vi "Teleop_TwistandDrive.vi"(9 "Joy Drive Input":dbl, 10 "Deadband X Value":dbl, 11 "Joy Twist Input":dbl) -> (3 "Twist Output":dbl[](array[numeric]))   [LabVIEW 2017]
panel:
  out "XY Graph":cluster{dbl[], dbl[]}(graph)
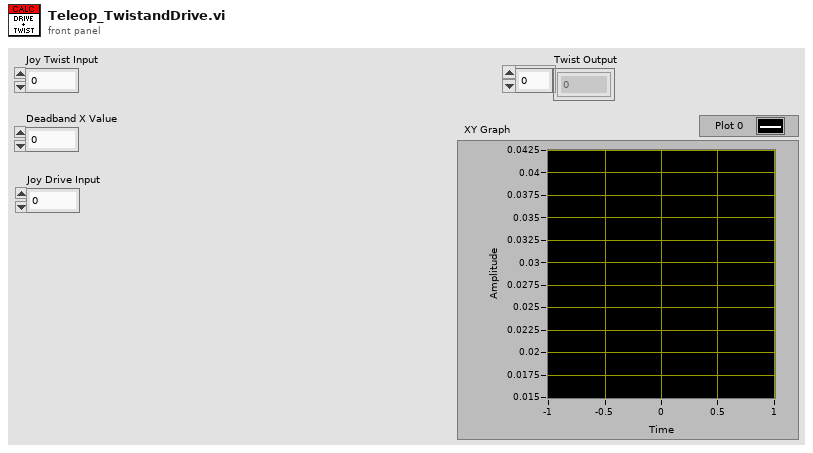
[diagram p1: front panel]
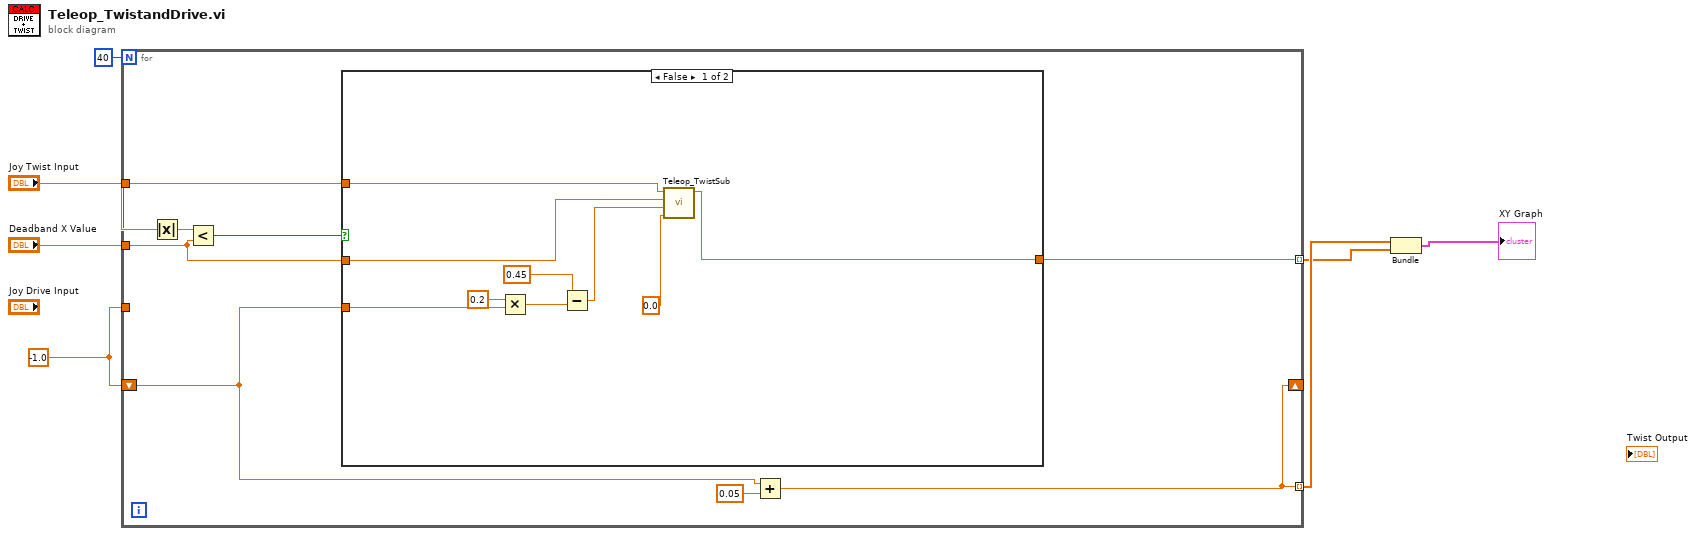
[diagram p0: block diagram]
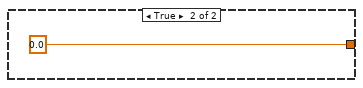
[diagram p2: hidden frame]
diagram:
  w1 = -1.0
  n1 = for {
    N: 40 -> [_]
    tunnel: "Joy Twist Input" -> [w13]
    tunnel: "Deadband X Value" -> [w12]
    tunnel: w1 -> [_]
    shift-right: [w10] -> _
    shift-left: w1 -> [w8]
    tunnel: [w10] -> w5 mode=indexing
    tunnel: [w9] -> w4 mode=indexing
    n2 = Absolute Value(x=w13) -> (abs(x)=w15:dbl)
    n3 = Less?(x=w15, y=w12) -> (x < y?=w14:bool)
    n4 = case shown="False" w14 {
      tunnel: [w23 0.0] -> w9
      tunnel: w13 -> [w24 _]
      tunnel: w12 -> [w22 _]
      tunnel: w8 -> [w20 _]
      frame False {
        n5 = Multiply(x=0.2, y=w20) -> (x*y=w19:dbl)
        n6 = Subtract(x=0.45, y=w19) -> (x-y=w17:dbl)
        n7 = call "Teleop_TwistSub.vi"("b - value"=0.0, "Scale Factor"=w17, "Deadband X value"=w22, "Input Twist"=w24) -> ("Twist Output"=w23:dbl)  [unwired: 7 in]
      }
      frame True {
      }
    }
    n8 = Add(x=w8, y=0.05) -> (x+y=w10:dbl)
  }
  n9 = Bundle(w5, w4) -> (→"XY Graph":cluster{dbl[], dbl[]})  [unwired: 1 in]
